vi "FisherPaykel Motor Setup 1.vi"(7 "Debug":bool, 8 "error in (no error)":errorcluster, 9 "Command Modifier":T1="0", 10 "Main Command":T2=">CS", 11 "VISA Refnum in":refnum<visa-resource-name>) -> (0 "error out":errorcluster, 3 "VISA Refnum out":refnum<visa-resource-name>)   [LabVIEW 2016]
uses:
  Type Definitions/Fisher Paykel Main Command.ctl
  Type Definitions/Checksum.ctl
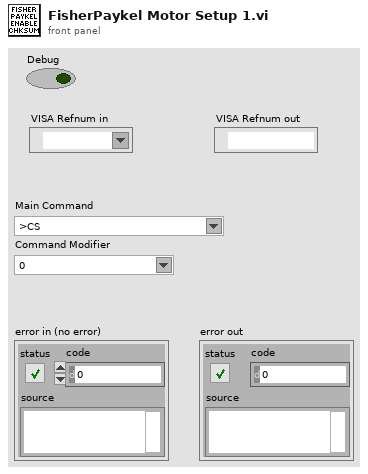
[diagram p1: front panel]
types:
  T1 = typedef "Checksum.ctl" = string
  T2 = typedef "Fisher Paykel Main Command.ctl" = string
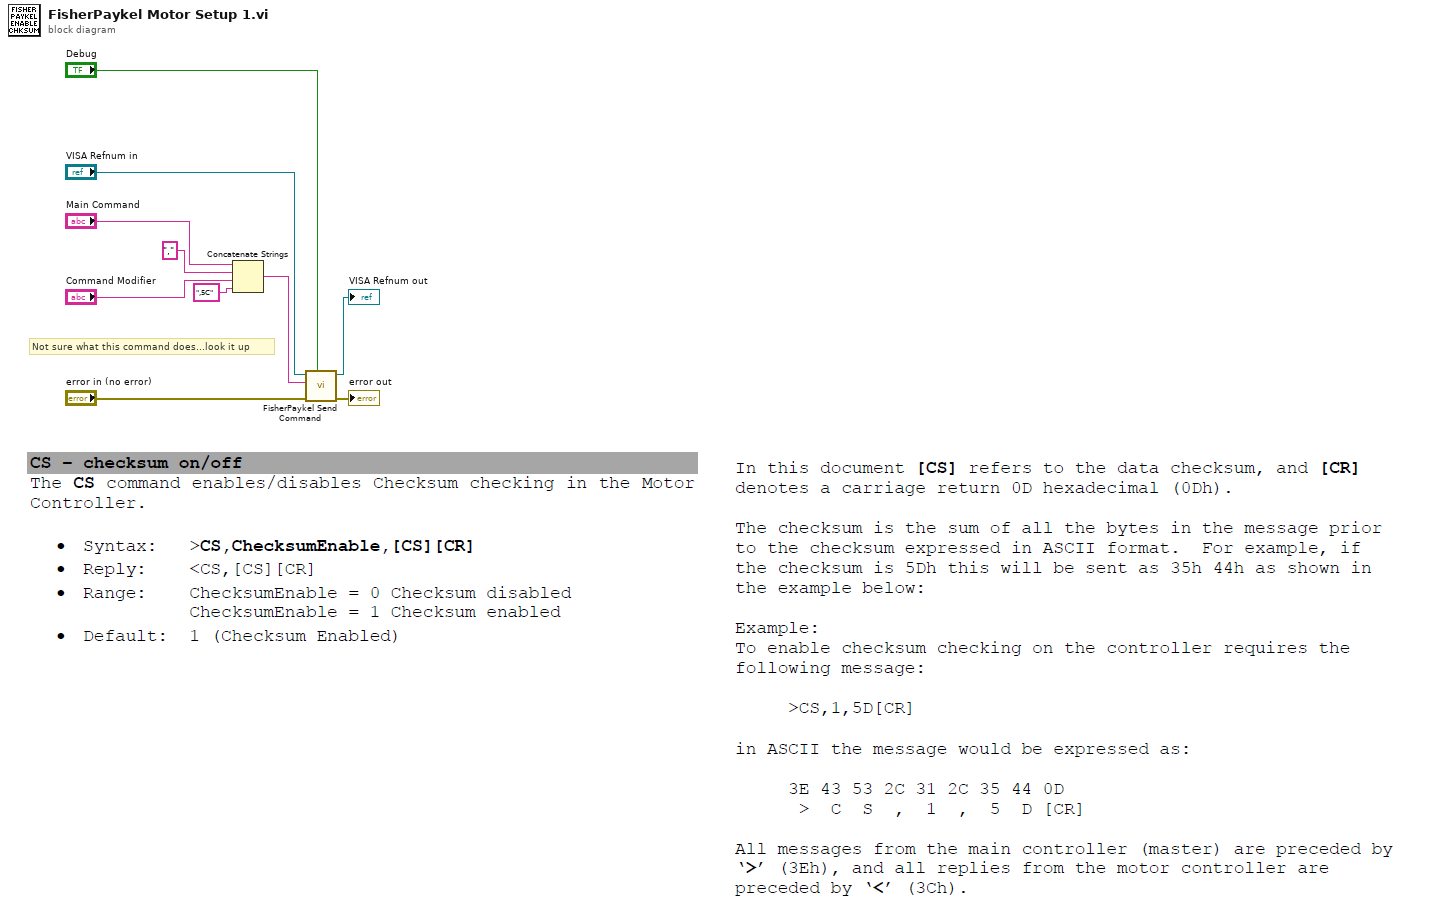
[diagram p0: block diagram]
diagram:
  # "Not sure what this command does...look it up"
  n1 = Concatenate Strings("Main Command", "," ("string"), "Command Modifier", ",5C" ("string")) -> (w6:string)
  n2 = call "FisherPaykel Send Command.vi"("Debug"="Debug", "error in (no error)"="error in (no error)", "Send Command"=w6, "VISA Refnum in"="VISA Refnum in") -> ("error out"=→"error out":errorcluster, "VISA Refnum out"=→"VISA Refnum out":refnum<visa-resource-name>)  [unwired: 5 in, 1 out]
